vi "ConfigDb.vi"(7 "EnableLog":bool, 9 "Event":T1={"obj_tag"="", "event_tag"="", "code"=enum."DI_RAW_LO", "Priority"=enum."Alert", "Value"=0.0, "Description"="", "Time Stamp"=timestamp(0 s since 1904-01-01)}, 10 "Logger":refnum<class "Logger.lvclass">, 11 "AnalogComparator in":refnum<class "AnalogComparator.lvclass">) -> (3 "AnalogComparator out":refnum<class "AnalogComparator.lvclass">)   [LabVIEW 2019, in "AnalogComparator.lvclass"]
uses:
  AnalogComparator.lvclass
  Logger_class/Logger.lvclass
  Logger_class/EventData.ctl
  Logger_class/EventCode.ctl
  Logger_class/Priority.ctl
  AnalogComparator.lvclass/AnalogComparator.ctl
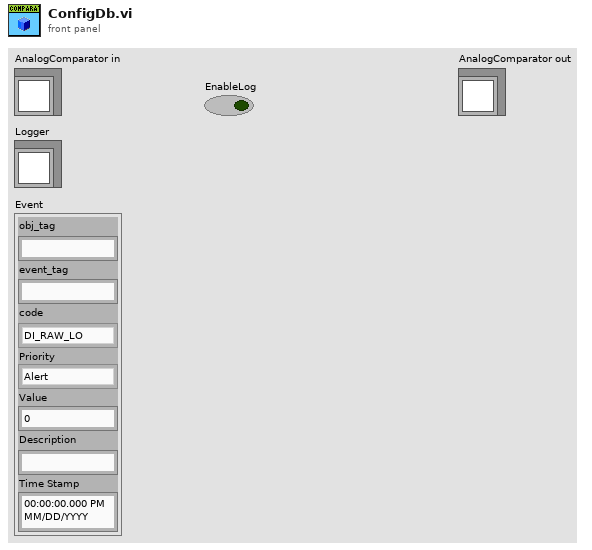
[diagram p1: front panel]
types:
  T1 = typedef "Logger.lvclass/EventData.ctl" = cluster{"obj_tag":string, "event_tag":string, "code":T2, "Priority":T3, "Value":dbl, "Description":string, "Time Stamp":timestamp}
  T2 = typedef "Logger.lvclass/EventCode.ctl" = enum16{"DI_EU_LO", "DI_EU_HI", "DIO_LO", "DIO_HI", "DI_RAW_LO", "DI_RAW_HI", "DO_LO", "DO_HI", "DA_OK", "DA_ALARM", "AA_HI", "AA_HIHI", "AA_LO", "AA_LOLO", "AA_OK", "CMD", "OUT_OF_RANGE_OK", "OUT_OF_RANGE_LO", "OUT_OF_RANGE_HI", "CONFIG", "DI_LO", "DI_HI"}
  T3 = typedef "Logger.lvclass/Priority.ctl" = enum16{"Alert", "Critical", "Error", "Warning", "Notice", "Informational", "Debug"}
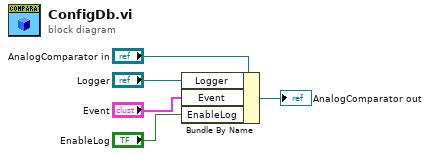
[diagram p0: block diagram]
diagram:
  n1 = Bundle By Name(cluster="AnalogComparator in", "Logger"="Logger", "Event"="Event", "EnableLog"="EnableLog") -> (→"AnalogComparator out":refnum<class "AnalogComparator.lvclass">)
